vi "VIP_Pre-Install Custom Action.vi"(10 "Variant":variant) -> (0 "error out":errorcluster)   [LabVIEW 2021]
uses:
  <vilib>/Utility/sysdir.llb/System Directory Type.ctl
  <userlib>/_OpenG.lib/file/file.llb/openg_file.lvlib
  <vilib>/Utility/config.llb/NI_LVConfig.lvlib
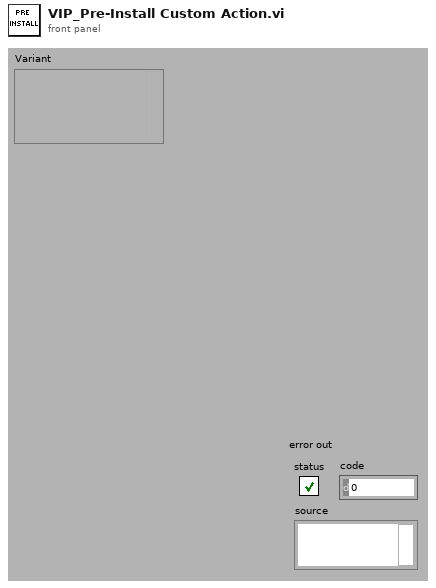
[diagram p1: front panel]
types:
  T1 = enum16{"open", "replace", "create", "open or create", "replace or create", "replace or create with confirmation"}
  T2 = typedef "System Directory Type.ctl" = i32
  T3 = typedef "NI_LVConfig.lvlib/Config Data RefNum.ctl" = refnum<k1>
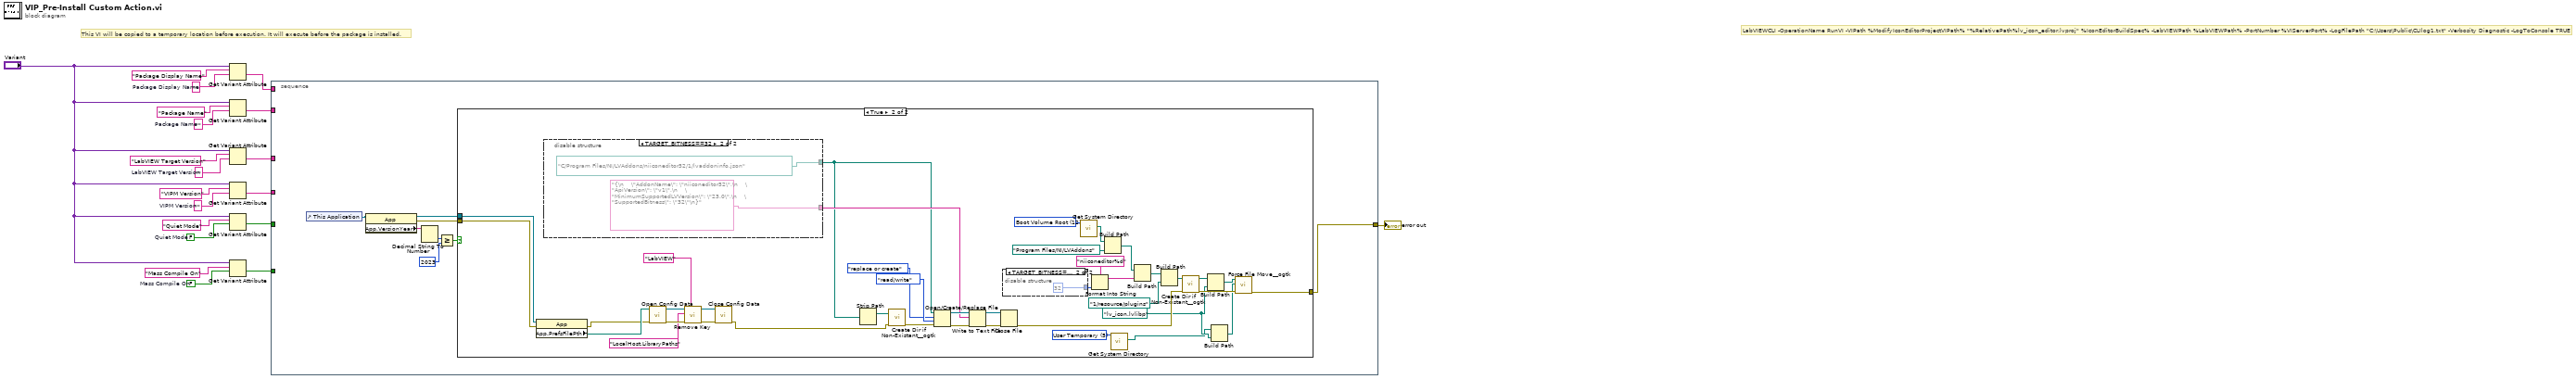
[diagram p0: block diagram]
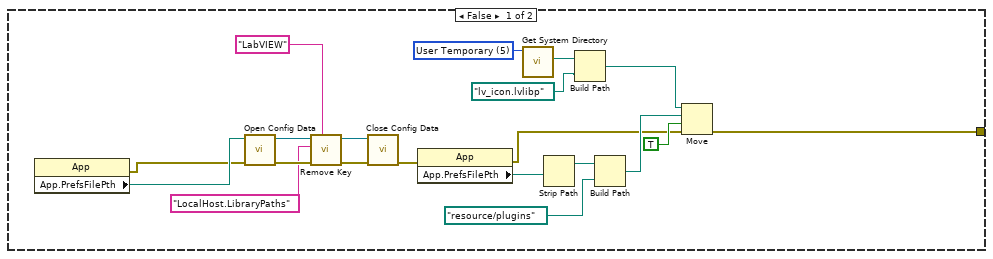
[diagram p2: hidden frame]
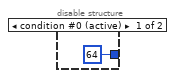
[diagram p3: hidden frame]
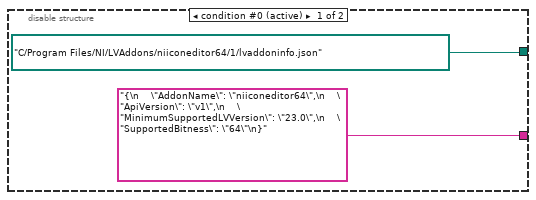
[diagram p4: hidden frame]
diagram:
  w2 = FALSE  # Mass Compile On
  w4 = ""  # Package Display Name
  w11 = FALSE  # Quiet Mode
  w14 = ""  # VIPM Version
  w16 = ""  # LabVIEW Target Version
  w18 = ""  # Package Name
  # "LabVIEWCLI -OperationName RunVI -VIPath %ModifyIconEditorProjectVIPath% \"%RelativePath%lv_icon_editor.lvproj\" %IconEditorBuildSpec% -LabVIEWPath %LabVIEWPath% -PortNumber %VIServerPort% -LogFilePath \"C:\\Users\\Public\\CLIlog1.txt\" -Verbosity Diagnostic -LogToConsole TRUE"
  # "This VI will be copied to a temporary location before execution. It will execute before the package is installed."
  n1 = Get Variant Attribute(Variant="Variant", name="Package Display Name", default value (empty Variant)=w4) -> (value=w10:string)  [unwired: 1 in, 3 out]
  n2 = Get Variant Attribute(Variant="Variant", name="Package Name", default value (empty Variant)=w18) -> (value=w9:string)  [unwired: 1 in, 3 out]
  n3 = Get Variant Attribute(Variant="Variant", name="LabVIEW Target Version", default value (empty Variant)=w16) -> (value=w8:string)  [unwired: 1 in, 3 out]
  n4 = Get Variant Attribute(Variant="Variant", name="VIPM Version", default value (empty Variant)=w14) -> (value=w7:string)  [unwired: 1 in, 3 out]
  n5 = Get Variant Attribute(Variant="Variant", name="Quiet Mode", default value (empty Variant)=w11) -> (value=w6:bool)  [unwired: 1 in, 3 out]
  n6 = Get Variant Attribute(Variant="Variant", name="Mass Compile On", default value (empty Variant)=w2) -> (value=w5:bool)  [unwired: 1 in, 3 out]
  n7 = stacked-sequence {
    tunnel: w10 -> [_]
    tunnel: w9 -> [_]
    tunnel: w8 -> [_]
    tunnel: w7 -> [_]
    tunnel: w6 -> [_]
    tunnel: w5 -> [_]
    tunnel: [w22] -> w1
    frame #0 {
      n8 = control-ref of="This Application"() -> (w28:refnum<vi>)
      n9 = property class="App"(reference=w28) -> (reference out=w21:refnum<vi>, error out=w23:errorcluster, "App.VersionYear"=w27:string)  [unwired: 1 in]
      n10 = Decimal String To Number(string=w27) -> (number=w26:i32)  [unwired: 2 in, 1 out]
      n11 = Greater Or Equal?(x=w26, y=2023) -> (x >= y?=w24:bool)
      n12 = case shown="True" w24 {
        tunnel: [w44 w88] -> w22
        tunnel: w23 -> [_ w50]
        tunnel: w21 -> [_ w49]
        frame False {
          w41 = T2 5 items=["User Home"=0, "User Desktop"=1, "User Documents"=2, "User Application Data"=3, "User Preferences"=4, "User Temporary"=5, "Public Documents"=6, "Public Application Data"=7, "Public Preferences"=8, "Public Cache"=13, "System Core Libraries"=9, "System Installed Libraries"=10, "Application Files"=11, "Boot Volume Root"=12] ("system directory type")
          n13 = property class="App"() -> (error out=w30:errorcluster, "App.PrefsFilePth"=w37:path)  [unwired: 2 in, 1 out]
          n14 = call <vilib>:"Open Config Data.vi"("error in (no error)"=w30, "configuration file path"=w37) -> ("error out"=w36:errorcluster, "refnum"=w34:T3)  [unwired: 7 in, 1 out]
          n15 = call <vilib>:"Remove Key.vi"("section"="LabVIEW", "error in (no error)"=w36, "key"="LocalHost.LibraryPaths", "refnum"=w34) -> ("error out"=w35:errorcluster, "refnum out"=w33:T3)  [unwired: 5 in, 1 out]
          n16 = call <vilib>:"Close Config Data.vi"("error in (no error)"=w35, "refnum"=w33) -> ("error out"=w29:errorcluster)  [unwired: 8 in, 1 out]
          n17 = property class="App"(error in=w29) -> (error out=w42:errorcluster, "App.PrefsFilePth"=w48:path)  [unwired: 1 in, 1 out]
          n18 = call <vilib>:"Get System Directory.vi"("system directory type"=w41) -> ("system directory"=w40:path)  [unwired: 10 in]
          n19 = Strip Path(path=w48) -> (stripped path=w47:path)  [unwired: 1 out]
          n20 = Build Path(base path=w40, name or relative path=path "lv_icon.lvlibp" ("source path")) -> (appended path=w38:path)
          n21 = Build Path(base path=w47, name or relative path=path "resource/plugins") -> (appended path=w45:path)
          n22 = Move(source path=w38, error in=w42, 9:TRUE ("overwrite (F)"), 10:w45) -> (error out=w44:errorcluster)  [unwired: 1 in, 2 out]
        }
        frame True {
          w52 = T2 5 items=["User Home"=0, "User Desktop"=1, "User Documents"=2, "User Application Data"=3, "User Preferences"=4, "User Temporary"=5, "Public Documents"=6, "Public Application Data"=7, "Public Preferences"=8, "Public Cache"=13, "System Core Libraries"=9, "System Installed Libraries"=10, "Application Files"=11, "Boot Volume Root"=12] ("system directory type")
          w65 = path "lv_icon.lvlibp" ("source path")
          w73 = T2 12 items=["User Home"=0, "User Desktop"=1, "User Documents"=2, "User Application Data"=3, "User Preferences"=4, "User Temporary"=5, "Public Documents"=6, "Public Application Data"=7, "Public Preferences"=8, "Public Cache"=13, "System Core Libraries"=9, "System Installed Libraries"=10, "Application Files"=11, "Boot Volume Root"=12] ("system directory type")
          n23 = property class="App"(reference=w49, error in=w50) -> (error out=w53:errorcluster, "App.PrefsFilePth"=w61:path)  [unwired: 1 out]
          n24 = disable-structure shown="TARGET_BITNESS==32" {
            disable-tunnel: [path "C:/Program Files/NI/LVAddons/niiconeditor64/1/lvaddoninfo.json" ("Destination[i] Paths (Absolute)") path "C:/Program Files/NI/LVAddons/niiconeditor32/1/lvaddoninfo.json" ("Destination[i] Paths (Absolute)")] -> w62
            disable-tunnel: ["{\n    \"AddonName\": \"niiconeditor64\",\n    \"ApiVersion\": \"v1\",\n    \"MinimumSupportedLVVersion\": \"23.0\",\n    \"SupportedBitness\": \"64\"\n}" ("Tag Name") "{\n    \"AddonName\": \"niiconeditor32\",\n    \"ApiVersion\": \"v1\",\n    \"MinimumSupportedLVVersion\": \"23.0\",\n    \"SupportedBitness\": \"32\"\n}" ("Tag Name")] -> w81
            frame condition #0 (active) {
            }
            frame condition #1 {
            }
          }
          n25 = call <vilib>:"Open Config Data.vi"("error in (no error)"=w53, "configuration file path"=w61) -> ("error out"=w60:errorcluster, "refnum"=w58:T3)  [unwired: 7 in, 1 out]
          n26 = call <vilib>:"Remove Key.vi"("section"="LabVIEW", "error in (no error)"=w60, "key"="LocalHost.LibraryPaths", "refnum"=w58) -> ("error out"=w59:errorcluster, "refnum out"=w57:T3)  [unwired: 5 in, 1 out]
          n27 = call <vilib>:"Close Config Data.vi"("error in (no error)"=w59, "refnum"=w57) -> ("error out"=w56:errorcluster)  [unwired: 8 in, 1 out]
          n28 = Strip Path(path=w62) -> (stripped path=w63:path)  [unwired: 1 out]
          n29 = call <userlib>:"Create Dir if Non-Existant__ogtk.vi"("error in (no error)"=w56, "Directory Path"=w63) -> ("error out"=w68:errorcluster)  [unwired: 7 in, 2 out]
          n30 = Open/Create/Replace File(file path (use dialog)=w62, error in=w68, operation (0:open)=T1."replace or create", access (0:read/write)=enum16{"read/write", "read-only", "write-only"}."read/write") -> (refnum out=w85:refnum<file>, error out=w86:errorcluster)  [unwired: 2 in, 1 out]
          n31 = Write to Text File(file (use dialog)=w85, text=w81, error in=w86) -> (refnum out=w84:refnum<file>, error out=w87:errorcluster)  [unwired: 1 in, 1 out]
          n32 = Close File(refnum=w84, error in=w87) -> (error out=w67:errorcluster)  [unwired: 1 out]
          n33 = disable-structure shown="TARGET_BITNESS==32" {
            disable-tunnel: [64 ("code") 32 ("code")] -> w76
            frame condition #0 (active) {
            }
            frame condition #1 {
            }
          }
          n34 = call <vilib>:"Get System Directory.vi"("system directory type"=w73) -> ("system directory"=w77:path)  [unwired: 10 in]
          n35 = Format Into String(format string="niiconeditor%d", w76) -> (resulting string=w79:string)  [unwired: 2 in, 1 out]
          n36 = Build Path(base path=w77, name or relative path=path "Program Files/NI/LVAddons") -> (appended path=w78:path)
          n37 = call <vilib>:"Get System Directory.vi"("system directory type"=w52) -> ("system directory"=w51:path)  [unwired: 10 in]
          n38 = Build Path(base path=w78, name or relative path=w79) -> (appended path=w80:path)
          n39 = Build Path(base path=w80, name or relative path=path "1/resource/plugins") -> (appended path=w71:path)
          n40 = call <userlib>:"Create Dir if Non-Existant__ogtk.vi"("error in (no error)"=w67, "Directory Path"=w71) -> ("error out"=w69:errorcluster, "dup Directory Path"=w70:path)  [unwired: 7 in, 1 out]
          n41 = Build Path(base path=w70, name or relative path=w65) -> (appended path=w66:path)
          n42 = Build Path(base path=w51, name or relative path=w65) -> (appended path=w64:path)
          n43 = call <userlib>:"Force File Move__ogtk.vi"("error in (no error)"=w69, "source"=w64, "target"=w66) -> ("error out"=w88:errorcluster)  [unwired: 3 in, 1 out]
        }
      }
    }
  }
  "error out" <- w1
